vi "Get Or Create Rfpm Switch Session.vi"(0 "logical name (\"SampleSwitch\")":string, 1 "option string (\"Simulate=0,RangeCheck=1,QueryInstrStatus=0,Cache=1\")":string="Simulate=0,RangeCheck=1,QueryInstrStatus=0,Cache=1", 11 "error in (no error)":errorcluster) -> (4 "Ivi Switch Session out":refnum<k15> caption="instrument handle out", 15 "error out":errorcluster)   [LabVIEW 2023, in "RFFixtureCharact.RFPM.lvlib" / "RF Subsystem Session Provider.lvclass"]
uses:
  RF Subsystem Session Provider.lvclass
  Common/Data Cache/Type Definitions/Dictionary Operation.ctl
  Common/RFCalAndFixtureCharact.Common.lvlib
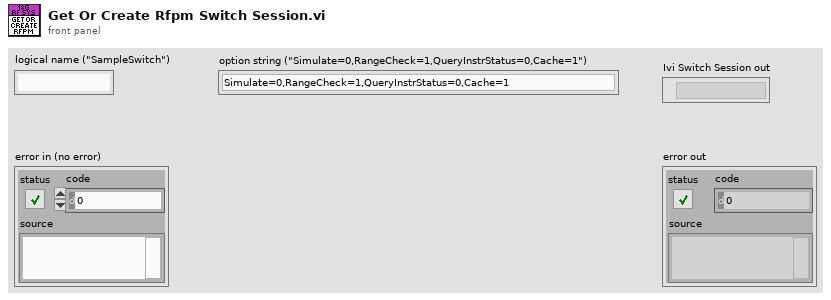
[diagram p1: front panel]
types:
  T1 = typedef "RFCalAndFixtureCharact.Common.lvlib/Dictionary Operation.ctl" = enum16{"Read", "Insert", "Remove", "Clear", "Get All", "Update"}
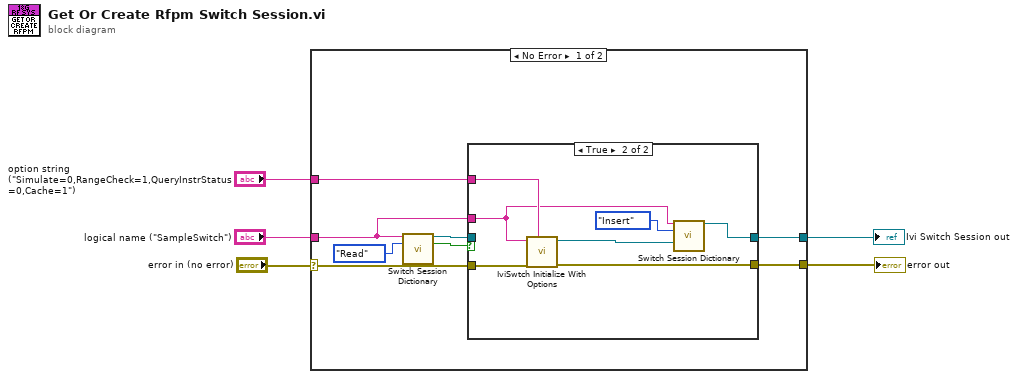
[diagram p0: block diagram]
diagram:
  n1 = case shown="No Error" "error in (no error)" {
    selector: "error in (no error)" -> [w9 w23]
    tunnel: "option string (\"Simulate=0,RangeCheck=1,QueryInstrStatus=0,Cache=1\")" -> [w11 _]
    tunnel: [w10 _] -> w4
    tunnel: [w7 w23] -> w2
    tunnel: "logical name (\"SampleSwitch\")" -> [w6 _]
    frame No Error {
      n2 = call "Switch Session Dictionary.vi"("Logical Name"=w6, "Action"=Dictionary_Operation."Read") -> ("Ivi Switch Session Out"=w8:refnum<k15>, "Switch session not found / already included"=w12:bool)  [unwired: 11 in, 1 out]
      n3 = case shown="True" w12 {
        tunnel: w11 -> [_ w22]
        tunnel: [w14 w18] -> w10
        tunnel: w9 -> [w15 w21]
        tunnel: w8 -> [w14 _]
        tunnel: [w15 w17] -> w7
        tunnel: w6 -> [_ w16]
        frame False {
        }
        frame True {
          n4 = call <vilib>:"IviSwtch Initialize With Options.vi"("option string (\"Simulate=0,RangeCheck=1,QueryInstrStatus=0,Cache=1\")"=w22, "error in (no error)"=w21, "logical name (\"SampleSwitch\")"=w16) -> ("error out"=w17:errorcluster, "instrument handle out"=w20:refnum<k15>)  [unwired: 7 in]
          n5 = call "Switch Session Dictionary.vi"("Logical Name"=w16, "Action"=Dictionary_Operation."Insert", "Ivi Switch Session In"=w20) -> ("Ivi Switch Session Out"=w18:refnum<k15>)  [unwired: 10 in, 2 out]
        }
      }
    }
    frame Error {
    }
  }
  "error out" <- w2
  "Ivi Switch Session out" <- w4
